vi "DVW_Read Array Waveform.vi"(3 "DVW Array":T1[](array[typedef])) -> (1 "Waveform Array":T2[](array[typedef]))   [LabVIEW 2020]
uses:
  Universal Controls/Waveform_Data.ctl
  TypeDefs_Utility/Ref_DVR_Buffer.ctl
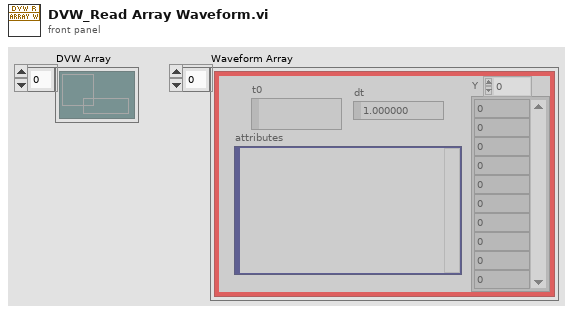
[diagram p1: front panel]
types:
  T1 = typedef "Ref_DVR_Buffer.ctl" = refnum<data-value>
  T2 = typedef "Waveform_Data.ctl" = waveform(dbl)
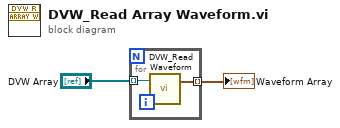
[diagram p0: block diagram]
diagram:
  n1 = for {
    tunnel: "DVW Array" -> [w4] mode=indexing
    tunnel: [w3] -> w2 mode=indexing
    n2 = call "DVW_Read Waveform.vi"("DVW"=w4) -> ("Raw Data Waveform Out"=w3:T2)  [unwired: 2 in]
  }
  "Waveform Array" <- w2
